vi "CaseStructure Get FrameNames.vi"(11 "GObject in":refnum<vi>) -> (1 "C code FrameNames":string[](array[string]), 2 "Frame Names":string[](array[string]), 3 "CaseSelector ref.":refnum<vi>)   [LabVIEW 2014]
doc: "Deal with CaseStructure FrameNames which should be cases in switch."
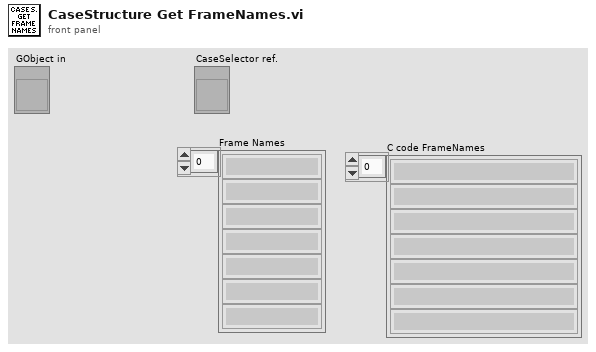
[diagram p1: front panel]
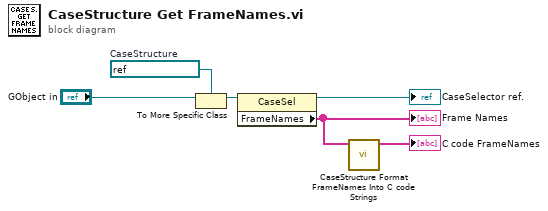
[diagram p0: block diagram]
diagram:
  w5 = refnum<vi> refnum  # CaseStructure
  n1 = To More Specific Class(target class=w5, reference="GObject in") -> (specific class reference=w6:refnum<vi>)  [unwired: 1 in, 1 out]
  n2 = property class="CaseSel"(reference=w6) -> (reference out=→"CaseSelector ref.":refnum<vi>, "FrameNames"=w2:string[])  [unwired: 1 in, 1 out]
  "Frame Names" <- w2
  n3 = call "CaseStructure Format FrameNames Into C code Strings.vi"("FrameNames in"=w2) -> ("c code cases names"=→"C code FrameNames":string[])  [unwired: 10 in]
